vi "Sleep for T_Out.vi"(6 "Disable FIFO Out Benchmark":bool, 7 "Convert External Clocks (T)":bool=TRUE, 8 "error in (no error)":errorcluster, 9 "Wake Offset (2000 ns)":i64=2000, 10 "T_Out (ns)":i64, 11 "CIFCorePlugin in":refnum<class "CIFCorePlugin.lvclass">) -> (0 "error out":errorcluster, 2 "T_Out Sleep Stats":T1, 3 "CIFCorePlugin out":refnum<class "CIFCorePlugin.lvclass">, 5 "Timeout (Housekeep now)":bool)   [LabVIEW 2021, in "CIFCorePlugin.lvclass"]
doc: "Physical outputs may be software timed. This will sleep until the requested T_Out time. It will wake early to allow time for driver processing according to the \"Wake Offset\" input. \n\nIf housekeeping is required before the requested T_Out it will wake early and set the Timeout to true, indicating T_Out should not be processed and instead housekeeping should occur.\n\nThis will also adjust for external clocks used in T_Out. This is typically used when outputting synchronized data to a DUT with an independent clock that is being tracked in the system. \n - If \"ClockID\" for the plugin is not zero \nAND\n - \"Plugin Timing Source\" for the plugin is True \nAND \n - \"Convert External Clocks\" input is True (default)\nT_Out will be converted from an external clock. \n\nThis will also Disable Auto Benchmarks for the plugin and record the timestamps for sleep and execute. The \"Benchmark Execute.VI\" should be called at the end of the execution step if this sleep is called. \n\nDisable FIFO Out Benchmark will disable automatic tracking of output error statistics."
uses:
  CIFCorePlugin.lvclass
  CIFCorePlugin.lvclass/CIFCorePlugin.ctl
  <vilib>/CIF Foundation/CIF Utilities/Time/Time_CIF_U.lvlib
  <vilib>/CIF Foundation/CIF Utilities/Time/Typedef/Future Time Event Limits.ctl
  Typedef/Logic Sleep Stats.ctl
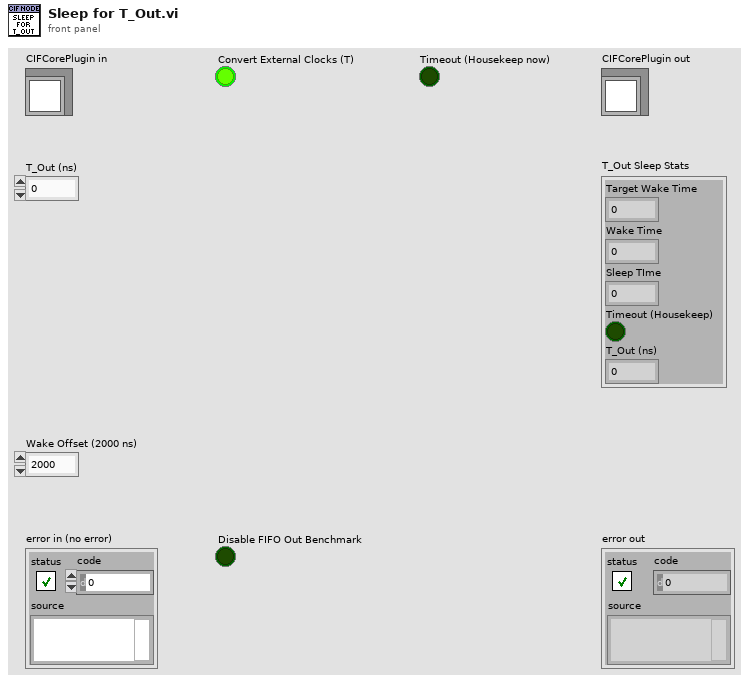
[diagram p1: front panel]
types:
  T1 = typedef "CIFCorePlugin.lvclass/Logic Sleep Stats.ctl" = cluster{"Target Wake Time":i64, "Wake Time":i64, "Sleep TIme":i64, "Timeout (Housekeep)":bool, "T_Out (ns)":i64}
  T2 = typedef "CIFCorePlugin.lvclass/Next Housekeep Times.ctl" = cluster{"Next Housekeep Time":i64, "Current Time (ns)":i64, "Time Until Next Housekeep (ns)":i64, "Time Until Next Housekeep (ms)":i64}
  T3 = typedef "Time_CIF_U.lvlib/Future Time Event Limits.ctl" = cluster{"Maximum":i64, "Minimum":i64}
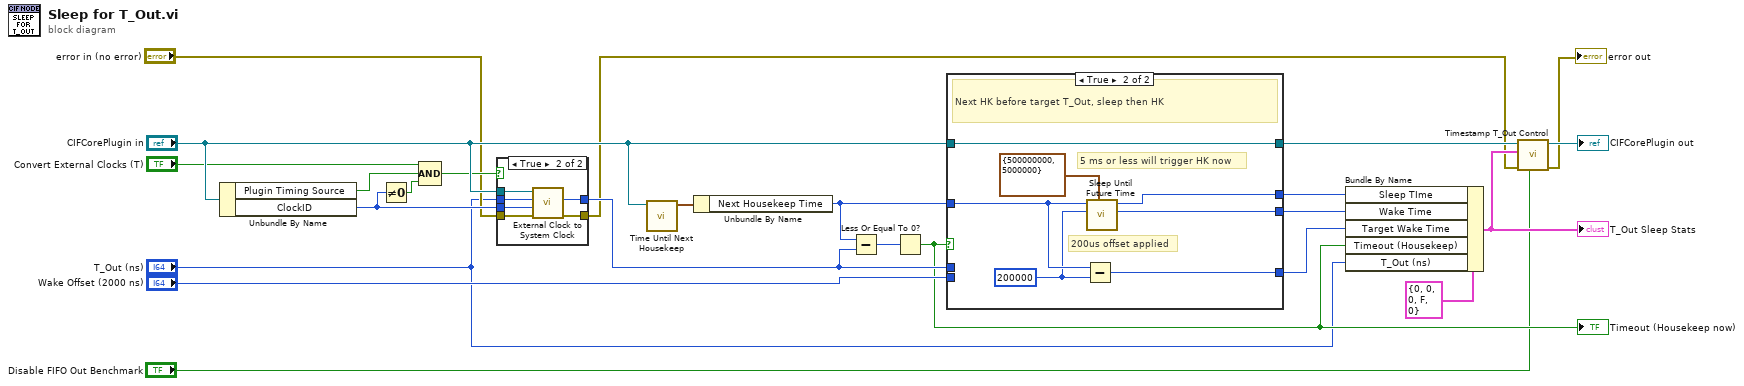
[diagram p0: block diagram]
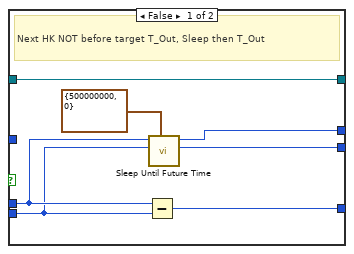
[diagram p2: hidden frame]
diagram:
  n1 = Unbundle By Name("CIFCorePlugin in") -> ("Plugin Timing Source"=w15:bool, "ClockID"=w20:u8)
  n2 = Not Equal To 0?(x=w20) -> (x != 0?=w19:bool)
  n3 = Compound Arithmetic op=AND("Convert External Clocks (T)", w15, w19) -> (w16:bool)
  n4 = case shown="True" w16 {
    tunnel: "T_Out (ns)" -> [w25 w32]
    tunnel: w20 -> [_ w31]
    tunnel: [w25 w30] -> w18
    tunnel: "CIFCorePlugin in" -> [_ w29]
    tunnel: "error in (no error)" -> [w26 w28]
    tunnel: [w26 w27] -> w4
    frame False {
    }
    frame True {
      n5 = call "External Clock to System Clock.vi"("error in (no error)"=w28, "ClockID"=w31, "External Time"=w32, "CIFCorePlugin in"=w29) -> ("error out"=w27:errorcluster, "System Time"=w30:i64)  [unwired: 4 in, 2 out]
    }
  }
  n6 = call "Time Until Next Housekeep.vi"("CIFCorePlugin in"="CIFCorePlugin in") -> ("Next Housekeep Times"=w22:T2)  [unwired: 9 in, 1 out]
  n7 = Unbundle By Name(w22) -> ("Next Housekeep Time"=w21:i64)
  n8 = Subtract(x=w21, y=w18) -> (x-y=w24:i64)
  n9 = Less Or Equal To 0?(x=w24) -> (x <= 0?=w8:bool)
  "Timeout (Housekeep now)" <- w8
  n10 = case shown="True" w8 {
    tunnel: w21 -> [_ w44]
    tunnel: w18 -> [w37 _]
    tunnel: "Wake Offset (2000 ns)" -> [w36 _]
    tunnel: [w34 w41] -> w7
    tunnel: "CIFCorePlugin in" -> [w34 w41]
    tunnel: [w38 w45] -> w10
    tunnel: [w33 w40] -> w11
    tunnel: [w35 w42] -> w9
    frame False {
      # "Next HK NOT before target T_Out, Sleep then T_Out"
      n11 = Subtract(x=w37, y=w36) -> (x-y=w35:i64)
      n12 = call <vilib>:"Sleep Until Future Time.vi"("FTE Limits (ns)"=T3 {"Maximum"=500000000, "Minimum"=0}, "Wake Offset"=w36, "Wake Time (ns)"=w37) -> ("Wake Time (ns)"=w38:i64, "Sleep TIme"=w33:i64)  [unwired: 6 in, 1 out]
    }
    frame True {
      w43 = i64 200000 ("Wake Offset")
      # "200us offset applied"
      # "5 ms or less will trigger HK now"
      # "Next HK before target T_Out, sleep then HK"
      n13 = Subtract(x=w44, y=w43) -> (x-y=w42:i64)
      n14 = call <vilib>:"Sleep Until Future Time.vi"("FTE Limits (ns)"=T3 {"Maximum"=500000000, "Minimum"=5000000}, "Wake Offset"=w43, "Wake Time (ns)"=w44) -> ("Wake Time (ns)"=w45:i64, "Sleep TIme"=w40:i64)  [unwired: 6 in, 1 out]
    }
  }
  n15 = Bundle By Name(cluster=T1 {"Target Wake Time"=0, "Wake Time"=0, "Sleep TIme"=0, "Timeout (Housekeep)"=FALSE, "T_Out (ns)"=0} ("Sleep Stats"), "Sleep TIme"=w11, "Wake Time"=w10, "Target Wake Time"=w9, "Timeout (Housekeep)"=w8, "T_Out (ns)"="T_Out (ns)") -> (w5:T1)
  "T_Out Sleep Stats" <- w5
  n16 = call "Timestamp T_Out Control.vi"("Disable FIFO Out Benchmark"="Disable FIFO Out Benchmark", "error in (no error)"=w4, "Logic Sleep Stats"=w5, "CIFCorePlugin in"=w7) -> ("error out"=→"error out":errorcluster, "CIFCorePlugin out"=→"CIFCorePlugin out":refnum<class "CIFCorePlugin.lvclass">)  [unwired: 6 in]
